vi "Summarize Project Items.vi"(9 "Member Data":string[][](array[string]), 11 "Project Summary":T1) -> (3 "Project Summary Out":T1)   [LabVIEW 2014]
uses:
  Type Defs/TYPE_Project Summary.ctl
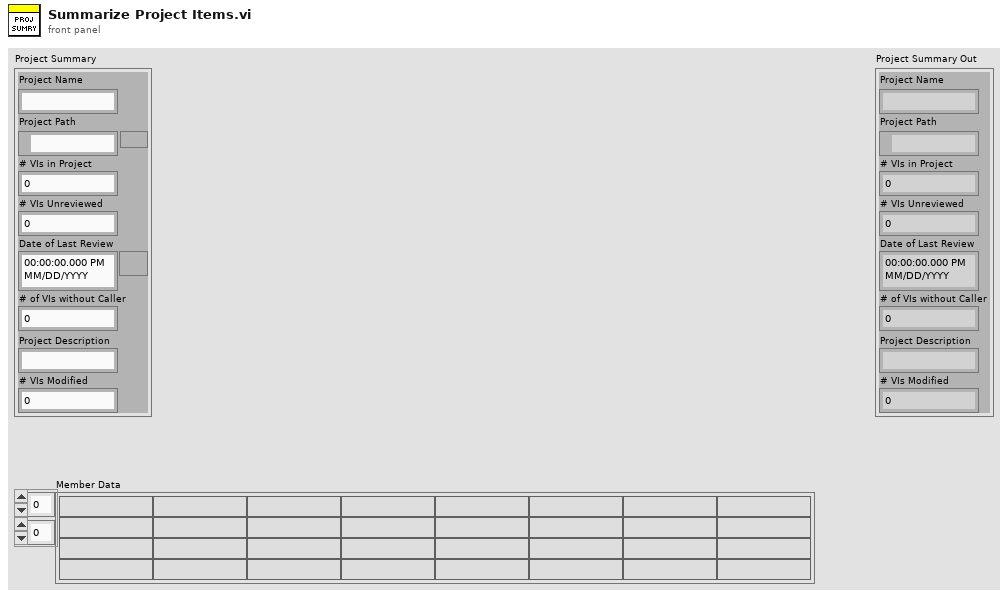
[diagram p1: front panel]
types:
  T1 = typedef "TYPE_Project Summary.ctl" = cluster{"Project Name":string, "Project Path":path, "# VIs in Project":i32, "# VIs Unreviewed":i32, "Date of Last Review":timestamp, "# of VIs without Caller":i32, "Project Description":string, "# VIs Modified":i32}
  T2 = typedef "TYPE_Version Status.ctl" = enum16{"Development", "alpha", "beta", "Reviewed", "Bug", "Other"}
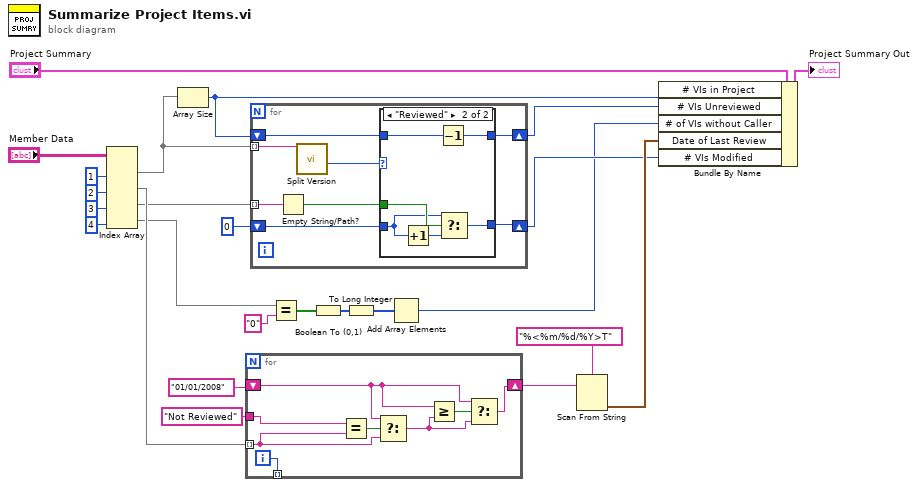
[diagram p0: block diagram]
diagram:
  n1 = Index Array(array="Member Data", index (col) #1=1 ("index (row)"), index (col) #2=2 ("index (col)"), index (col) #3=3 ("index (col)"), index (col) #4=4 ("index (col)")) -> (element #1=w21:string[], element #2=w12:string[], element #3=w10:string[], element #4=w6:string[])  [unwired: 4 in]
  n2 = Array Size(array=w21) -> (size(s)=w19:i32)
  n3 = for {
    shift-right: [w32] -> w18
    shift-left: "01/01/2008" ("y") -> [w29]
    tunnel: w12 -> [w26] mode=indexing
    tunnel: [w31] -> _ mode=indexing
    tunnel: "Not Reviewed" -> [w27]
    i -> [w31]
    n4 = Equal?(x=w27, y=w26) -> (x = y?=w30:bool)
    n5 = Select(t=w29, s=w30, f=w26) -> (s? t:f=w28:string)
    n6 = Greater Or Equal?(x=w29, y=w28) -> (x >= y?=w33:bool)
    n7 = Select(t=w29, s=w33, f=w28) -> (s? t:f=w32:string)
  }
  n8 = for {
    tunnel: w21 -> [w39] mode=indexing
    shift-right: [w41] -> w20
    shift-left: w19 -> [w40]
    tunnel: w10 -> [w38] mode=indexing
    shift-right: [w35] -> w8
    shift-left: 0 ("size(s)") -> [w36]
    n9 = Empty String/Path?(string/path=w38) -> (empty?=w37:bool)
    n10 = call <userlib>:"Split Version.vi"("VI Version"=w39) -> ("Current Phase"=w34:T2)  [unwired: 7 in, 3 out]
    n11 = case shown="\"Reviewed\"" w34 {
      tunnel: [w43 w49] -> w41
      tunnel: w40 -> [w43 w48]
      tunnel: w37 -> [_ w47]
      tunnel: w36 -> [w42 w45]
      tunnel: [w42 w46] -> w35
      frame Default {
      }
      frame "Reviewed" {
        n12 = Increment(x=w45) -> (x+1=w44:i32)
        n13 = Decrement(x=w48) -> (x-1=w49:i32)
        n14 = Select(t=w45, s=w47, f=w44) -> (s? t:f=w46:i32)
      }
    }
  }
  n15 = Equal?(x=w6, y="0") -> (x = y?=w4:bool[])
  n16 = Boolean To (0,1)(Boolean=w4) -> (0, 1=w3:i16[])
  n17 = To Long Integer(number=w3) -> (32bit integer=w1:i32[])
  n18 = Add Array Elements(numeric array=w1) -> (sum=w2:i32)
  n19 = Scan From String(format string="%<%m/%d/%Y>T", input string=w18) -> (output 1=w16:timestamp)  [unwired: 3 in, 3 out]
  n20 = Bundle By Name(cluster="Project Summary", "# VIs in Project"=w19, "# VIs Unreviewed"=w20, "# of VIs without Caller"=w2, "Date of Last Review"=w16, "# VIs Modified"=w8) -> (→"Project Summary Out":T1)
